vi "example_02_extract.vi"() -> ()   [LabVIEW 2015, in "lv-bin-7zip.lvlib" / "v1.lvlib"]
uses:
  v1.lvlib
  <userlib>/antonio-alexander/lv-bin/lv-bin/public/api/v1/advanced/add_data_path_multiple.vi
  advanced/extract_exe_archive.vi
  <userlib>/antonio-alexander/lv-bin/lv-bin/public/api/v1/v1.lvlib
panel:
  out "target_path out":path
  out "archive_path out":path
  out "files []":path[](array[path])
  out "error out":errorcluster
  in  "target_path in":path
  in  "archive_path":path
  in  "preview?":bool
  in  "bin_path":path
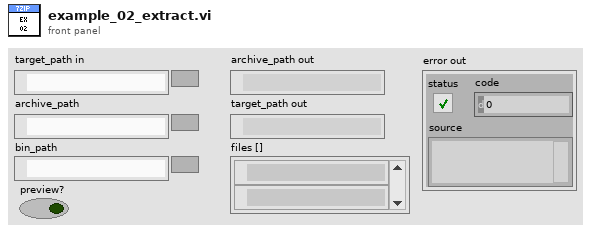
[diagram p1: front panel]
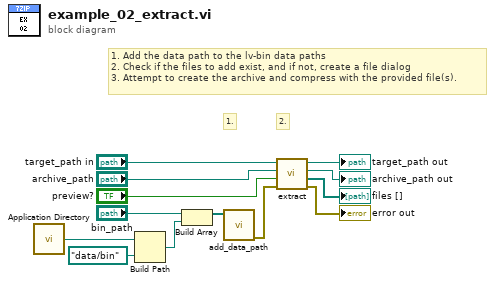
[diagram p0: block diagram]
diagram:
  # "1."
  # "1. Add the data path to the lv-bin data paths\n2. Check if the files to add exist, and if not, create a file dialog\n3. Attempt to create the archive and compress with the provided file(s)."
  # "2."
  n1 = call <vilib>:"Application Directory.vi"() -> ("Application Directory"=w10:path)
  n2 = Build Path(base path=w10, name or relative path=path "data/bin" ("Application Directory")) -> (appended path=w11:path)
  n3 = Build Array("bin_path", w11) -> (w12:path[])
  n4 = call-poly <userlib>:"add_data_path.vi"("path_to_add []"=w12) -> ("error out"=w8:errorcluster)  [unwired: 10 in]
  n5 = call-poly "extract.vi"("error in (no error)"=w8, "preview?"="preview?", "archive_path"="archive_path", "target_path in"="target_path in") -> ("error out"=→"error out":errorcluster, "files []"=→"files []":path[], "archive_path out"=→"archive_path out":path, "target_path out"=→"target_path out":path)  [unwired: 4 in]
